vi "Convert .NET Error to LabVIEW Error.vi"(8 "error in":errorcluster, 11 ".NET Refnum in":refnum<k39>) -> (0 "error out":errorcluster)   [LabVIEW 2027, in "Runtime Configuration File API.lvlib"]
uses:
  Runtime Configuration File API.lvlib
  C:/NetCoreDLL/NationalInstruments.VeriStand.dll
  NetCoreDLL/NationalInstruments.VeriStand.dll
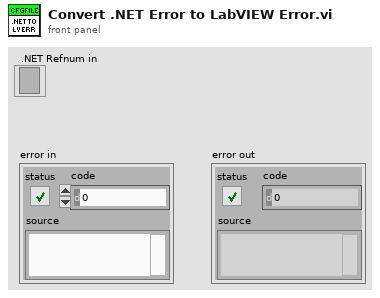
[diagram p1: front panel]
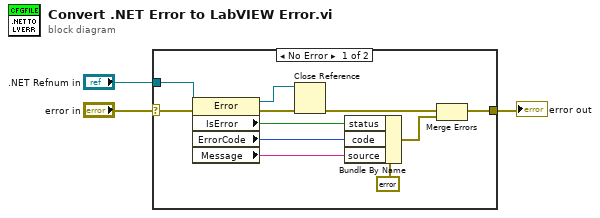
[diagram p0: block diagram]
diagram:
  n1 = case shown="No Error" "error in" {
    selector: "error in" -> [w9 w15]
    tunnel: ".NET Refnum in" -> [w4 _]
    tunnel: [w12 w15] -> w3
    frame No Error {
      n2 = property class="Error"(reference=w4, error in=w9) -> (reference out=w8:refnum<k39>, error out=w13:errorcluster, "IsError"=w5:bool, "ErrorCode"=w6:i32, "Message"=w7:string)
      n3 = Close Reference(reference=w8, error in (no error)=w13) -> (error out=w14:errorcluster)
      n4 = Bundle By Name(cluster=errorcluster {"status"=FALSE, "code"=0, "source"=""} ("error in (no error)"), "status"=w5, "code"=w6, "source"=w7) -> (w11:errorcluster)
      n5 = Merge Errors(w14, w11) -> (w12:errorcluster)
    }
    frame Error {
    }
  }
  "error out" <- w3
